vi "test_polymorphic_VI.vi"() -> ()   [LabVIEW 2020]
uses:
  created_VI/10_10_Fxp_addation.vi
panel:
  out "x+y":fxp<+/-,11,11>
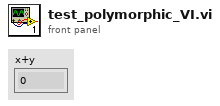
[diagram p1: front panel]
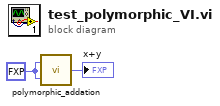
[diagram p0: block diagram]
diagram:
  w2 = fxp<+/-,10,10> 1.0
  n1 = call-poly "polymorphic_addation.vi"("y"=w2, "x"=w2) -> ("x+y"=→"x+y":fxp<+/-,11,11>)
